vi "ReportServices.vi"(1 "Destination":T4={"Subsystem Id"=42, "Node Id"=1, "Component Id"=1}, 2 "NodeList":T1[](array[typedef])=[{"Node Id"=1, "ComponentSeq"=[{"Component Id"=1, "Instance Id"=0, "ServiceSeq"=[{"ServiceURI"="ListManager", "MajorVerNum"=1, "MinorVerNum"=0}, {"ServiceURI"="Management", "MajorVerNum"=1, "MinorVerNum"=0}, {"ServiceURI"="LocalWaypointListDriver", "MajorVerNum"=1, "MinorVerNum"=0}, {"ServiceURI"="LocalPoseSensor", "MajorVerNum"=1, "MinorVerNum"=0}, {"ServiceURI"="AccessControl", "MajorVerNum"=1, "MinorVerNum"=0}, {"ServiceURI"="Discovery", "MajorVerNum"=1, "MinorVerNum"=0}, {"ServiceURI"="VelocityStateSensor", "MajorVerNum"=1, "MinorVerNum"=0}]}]}], 3 "Source":T4={"Subsystem Id"=221, "Node Id"=1, "Component Id"=1}) -> (0 "Encoded JAUS Message":string)   [LabVIEW 2009]
uses:
  Support Files/Address.ctl
  Support Files/NodeRec.ctl
  Support Files/ComponentRec.ctl
  Support Files/ServiceRec.ctl
panel:
  in  "Command Code":string="K\u0003"
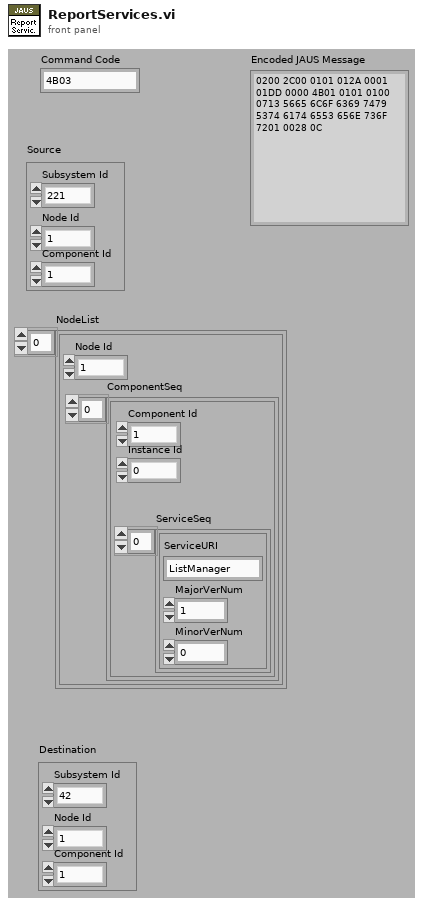
[diagram p1: front panel]
types:
  T1 = typedef "NodeRec.ctl" = cluster{"Node Id":u8, "ComponentSeq":T2[]}
  T2 = typedef "ComponentRec.ctl" = cluster{"Component Id":u8, "Instance Id":u8, "ServiceSeq":T3[]}
  T3 = typedef "ServiceRec.ctl" = cluster{"ServiceURI":string, "MajorVerNum":u8, "MinorVerNum":u8}
  T4 = typedef "Address.ctl" = cluster{"Subsystem Id":u16, "Node Id":u8, "Component Id":u8}
  T5 = cluster{"unsigned byte array[0]":u8, "unsigned byte array[1]":u8}
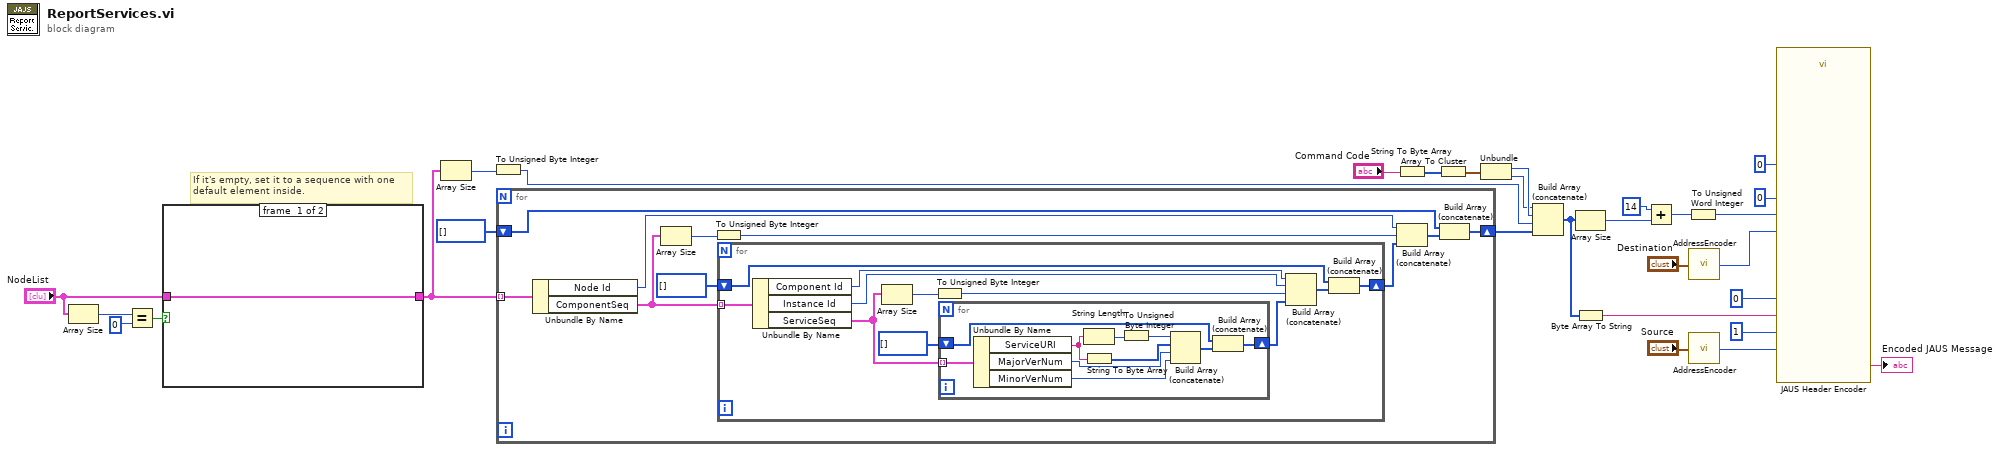
[diagram p0: block diagram]
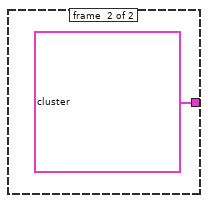
[diagram p2: hidden frame]
diagram:
  # "If it's empty, set it to a sequence with one \ndefault element inside."
  n1 = Array Size(array="NodeList") -> (size(s)=w7:i32)
  n2 = Equal?(x=w7, y=0) -> (x = y?=w5:bool)
  n3 = case shown="False" w5 {
    tunnel: [w30 T1[] [{"Node Id"=1, "ComponentSeq"=[{"Component Id"=1, "Instance Id"=0, "ServiceSeq"=[{"ServiceURI"="Service", "MajorVerNum"=1, "MinorVerNum"=1}]}]}] ("NodeList")] -> w3
    tunnel: "NodeList" -> [w30 _]
    frame #0 {
    }
    frame #1 {
    }
  }
  n4 = Array Size(array=w3) -> (size(s)=w16:i32)
  n5 = To Unsigned Byte Integer(number=w16) -> (unsigned 8bit integer=w8:u8)
  n6 = for {
    tunnel: w3 -> [w41] mode=indexing
    shift-right: [w32] -> w1
    shift-left: u8[] [] -> [w35]
    n7 = Unbundle By Name(w41) -> ("Node Id"=w40:u8, "ComponentSeq"=w39:T2[])
    n8 = Array Size(array=w39) -> (size(s)=w38:i32)
    n9 = To Unsigned Byte Integer(number=w38) -> (unsigned 8bit integer=w37:u8)
    n10 = for {
      tunnel: w39 -> [w52] mode=indexing
      shift-right: [w44] -> w33
      shift-left: u8[] [] -> [w46]
      n11 = Unbundle By Name(w52) -> ("Component Id"=w51:u8, "Instance Id"=w50:u8, "ServiceSeq"=w49:T3[])
      n12 = Array Size(array=w49) -> (size(s)=w48:i32)
      n13 = To Unsigned Byte Integer(number=w48) -> (unsigned 8bit integer=w47:u8)
      n14 = for {
        tunnel: w49 -> [w62] mode=indexing
        shift-right: [w53] -> w42
        shift-left: u8[] [] -> [w55]
        n15 = Unbundle By Name(w62) -> ("ServiceURI"=w60:string, "MajorVerNum"=w58:u8, "MinorVerNum"=w57:u8)
        n16 = String Length(string=w60) -> (length=w61:i32)
        n17 = String To Byte Array(string=w60) -> (unsigned byte array=w59:u8[])
        n18 = To Unsigned Byte Integer(number=w61) -> (unsigned 8bit integer=w56:u8)
        n19 = Build Array (concatenate)(w56, w59, w58, w57) -> (w54:u8[])
        n20 = Build Array (concatenate)(w55, w54) -> (w53:u8[])
      }
      n21 = Build Array (concatenate)(w51, w50, w47, w42) -> (w45:u8[])
      n22 = Build Array (concatenate)(w46, w45) -> (w44:u8[])
    }
    n23 = Build Array (concatenate)(w40, w37, w33) -> (w34:u8[])
    n24 = Build Array (concatenate)(w35, w34) -> (w32:u8[])
  }
  n25 = String To Byte Array(string="Command Code") -> (unsigned byte array=w20:u8[])
  n26 = Array To Cluster(array=w20) -> (cluster=w19:T5)
  n27 = Unbundle(w19) -> ("unsigned byte array[0]"=w18:u8, "unsigned byte array[1]"=w17:u8)
  n28 = Build Array (concatenate)(w17, w18, w8, w1) -> (w15:u8[])
  n29 = Array Size(array=w15) -> (size(s)=w13:i32)
  n30 = Byte Array To String(unsigned byte array=w15) -> (string=w22:string)
  n31 = Add(x=14 ("Data Size (8-23)"), y=w13) -> (x+y=w12:i32)
  n32 = To Unsigned Word Integer(number=w12) -> (unsigned 16bit integer=w11:u16)
  n33 = call "AddressEncoder.vi"("Address Cluster"="Destination") -> ("Address"=w27:u32)
  n34 = call "AddressEncoder.vi"("Address Cluster"="Source") -> ("Address"=w28:u32)
  n35 = call "JAUS Header Encoder.vi"("Message Type (0-5)"=u8 0, "Data Size (8-23)"=w11, "Priority(40-41)"=u8 1, "Payload"=w22, "Source ID (80-95)"=w28, "Destination ID (48-79)"=w27, "Data Flags (46-47)"=u8 0, "Ack/Nak (44-45)"=u8 0) -> ("Encoded JAUS Message"=→"Encoded JAUS Message":string)  [unwired: 7 in]
